vi "CommandType2String.vi"(10 "Command\nType":enum16{"<None>", "Displacement", "Force"}[](array[ring])) -> (2 "String":string)   [LabVIEW 2009]
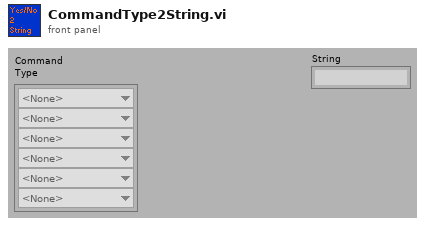
[diagram p1: front panel]
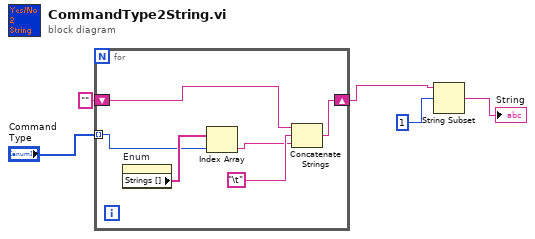
[diagram p0: block diagram]
diagram:
  n1 = for {
    shift-right: [w10] -> w4
    shift-left: "" -> [w11]
    tunnel: "Command\nType" -> [w7] mode=indexing
    n2 = property on="Enum" class="Enum (strict)"() -> ("Strings []"=w8:string[])  [unwired: 2 in, 2 out]
    n3 = Index Array(array=w8, index=w7) -> (element=w6:string)
    n4 = Concatenate Strings(w11, "\t", w6) -> (w10:string)
  }
  n5 = String Subset(string=w4, offset (0)=1) -> (substring=→"String":string)  [unwired: 1 out]
